vi "layout.vi"(0 "reference":refnum<class "UseCaseNode.lvclass">, 1 "graph":refnum<class "Graph.lvclass">, 2 "graphics":refnum<class "Graphics.lvclass">, 3 "grid":refnum<class "Grid.lvclass">, 5 "error in (no error)":errorcluster) -> (14 "reference out":refnum<class "UseCaseNode.lvclass">, 19 "error out":errorcluster)   [LabVIEW 2014, in "UseCaseNode.lvclass"]
doc: "public void layout(Graph g, Graphics2D g2, Grid grid)"
uses:
  <resource>/Framework/Providers/Open_GDS/UML/UseCaseNode_class/UseCaseNode.lvclass
  <resource>/Framework/Providers/Open_GDS/UML/Graph_class/Graph.lvclass
  <resource>/Framework/Providers/Open_GDS/UML/Graphics_class/Graphics.lvclass
  <resource>/Framework/Providers/Open_GDS/UML/Grid_class/Grid.lvclass
  <resource>/Framework/Providers/Open_GDS/UML/General/Rectangle/Rectangle Rectangle2D.ctl
  <resource>/Framework/Providers/Open_GDS/UML/MultiLineString_class/MultiLineString.lvclass
  <resource>/Framework/Providers/Open_GDS/UML/RectangularNode_class/RectangularNode.lvclass
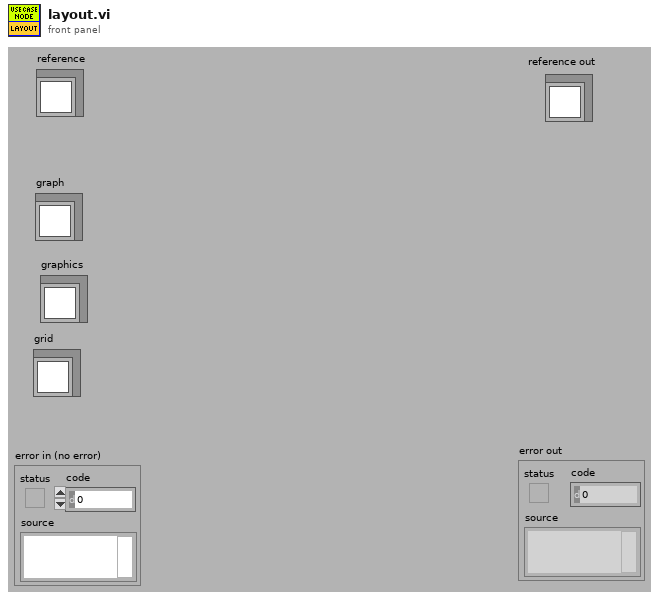
[diagram p1: front panel]
types:
  T1 = typedef "Rectangle Rectangle2D.ctl" = cluster{"x":dbl, "y":dbl, "width":dbl, "height":dbl}
  T2 = typedef "UseCaseNode.lvclass/ObjectAttributes.ctl" = cluster{"name":refnum<class "MultiLineString.lvclass">, "DEFAULT_WIDTH":i32, "DEFAULT_HEIGHT":i32}
  T3 = typedef "RectangularNode.lvclass/ObjectAttributes.ctl" = cluster{"bounds":T1}
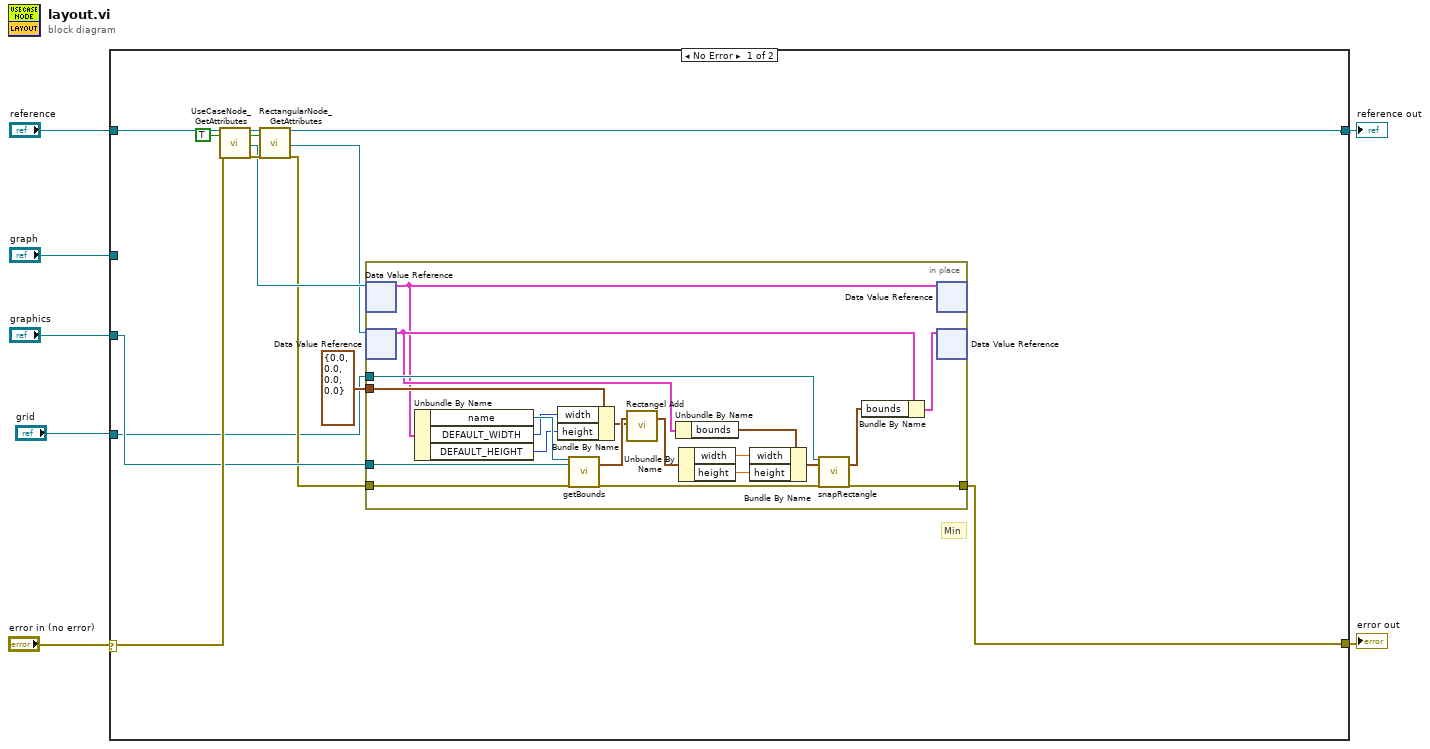
[diagram p0: block diagram]
diagram:
  n1 = case shown="No Error" "error in (no error)" {
    selector: "error in (no error)" -> [w18 w41]
    tunnel: "reference" -> [w20 w42]
    tunnel: [w9 w41] -> w6
    tunnel: [w19 w42] -> w5
    tunnel: "graph" -> [_ _]
    tunnel: "graphics" -> [w13 _]
    tunnel: "grid" -> [w10 _]
    frame No Error {
      w8 = TRUE ("OnlyGetDvrReference(False)")
      # "Min"
      n2 = call <resource>:"UseCaseNode_GetAttributes.vi"("reference in"=w20, "OnlyGetDvrReference(False)"=w8, "error in (no error)"=w18) -> ("reference out"=w17:refnum<class "UseCaseNode.lvclass">, "DataRef"=w15:refnum<data-value>, "error out"=w16:errorcluster)  [unwired: 13 in, 1 out]
      n3 = call <resource>:"RectangularNode_GetAttributes.vi"("reference in"=w17, "OnlyGetDvrReference(False)"=w8, "error in (no error)"=w16) -> ("reference out"=w19:refnum<class "UseCaseNode.lvclass">, "DataRef"=w14:refnum<data-value>, "error out"=w12:errorcluster)  [unwired: 13 in, 1 out]
      n4 = in-place {
        in-place-border: w13 -> [w37]
        in-place-border: w12 -> [w36]
        in-place-border: T1 {"x"=0.0, "y"=0.0, "width"=0.0, "height"=0.0} ("bounds") -> [w33]
        in-place-border: w10 -> [w30]
        in-place-border: [w27] -> w9
        n5 = in-place-dvr #1(w15) -> (w21:T2)  [unwired: 1 out]
        n6 = in-place-dvr #2(w14) -> (w23:T3)  [unwired: 1 out]
        n7 = Unbundle By Name(w21) -> ("name"=w40:refnum<class "MultiLineString.lvclass">, "DEFAULT_WIDTH"=w39:i32, "DEFAULT_HEIGHT"=w38:i32)
        n8 = Bundle By Name(cluster=w33, "width"=w39, "height"=w38) -> (w32:T1)
        n9 = call-dynamic "getBounds.vi"("reference"=w40, "graphics"=w37, "error in (no error)"=w36) -> ("bounds"=w35:T1, "error out"=w34:errorcluster)  [unwired: 15 out]
        n10 = call <resource>:"Rectangel Add.vi"("bounds1"=w35, "bounds2"=w32) -> ("boundsAdded"=w31:T1)  [unwired: 3 in, 14 out]
        n11 = Unbundle By Name(w23) -> ("bounds"=w24:T1)
        n12 = Unbundle By Name(w31) -> ("width"=w26:dbl, "height"=w25:dbl)
        n13 = Bundle By Name(cluster=w24, "width"=w26, "height"=w25) -> (w29:T1)
        n14 = call <resource>:"snapRectangle.vi"("reference"=w30, "bounds"=w29, "error in (no error)"=w34) -> ("boundsOut"=w28:T1, "error out"=w27:errorcluster)  [unwired: 15 out]
        n15 = Bundle By Name(cluster=w23, "bounds"=w28) -> (w22:T3)
        n16 = in-place-dvr #1(w21) -> ()  [unwired: 2 out]
        n17 = in-place-dvr #2(w22) -> ()  [unwired: 2 out]
      }
    }
    frame Error {
    }
  }
  "reference out" <- w5
  "error out" <- w6
